vi "Poehali.vi"() -> (0 "?":string)   [LabVIEW 2016]
uses:
  Global 3.vi
panel:
  in  "Back":bool
  in  "?":bool
  out "2D Picture":picture
  # "Nice to meet you,  here,"
  # "You are at the Diversity orbital station. Here you can learn, create , grow and just \"dive into\" space exploration.\n        \n       Hope you will have fun !"
  # "ARE YOU READY ?"
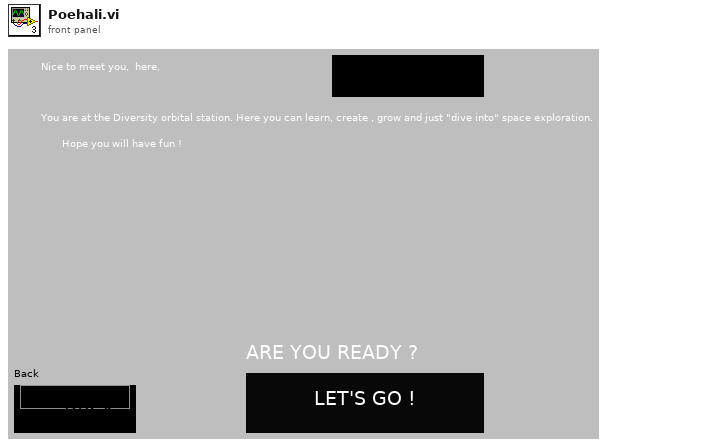
[diagram p1: front panel]
types:
  T1 = enum32{"Invalid", "Standard", "Closed", "Hidden", "Minimized", "Maximized"}
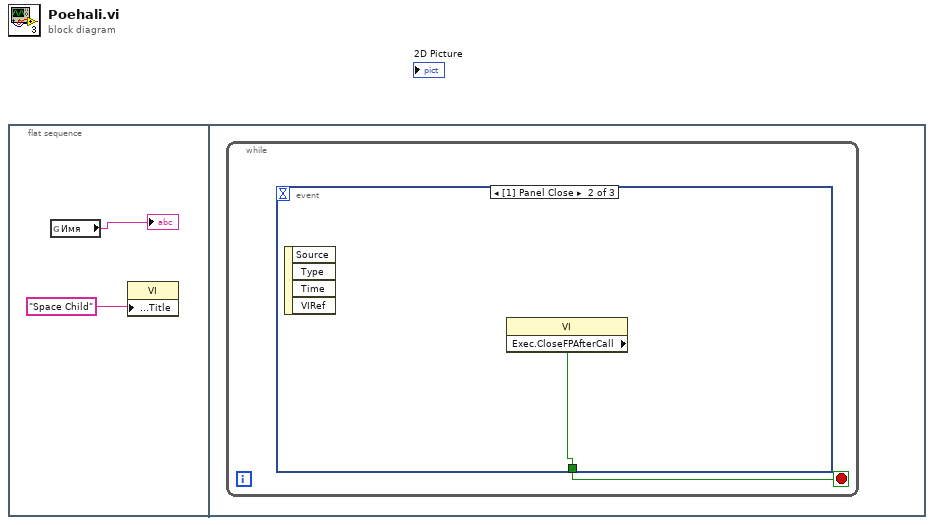
[diagram p0: block diagram]
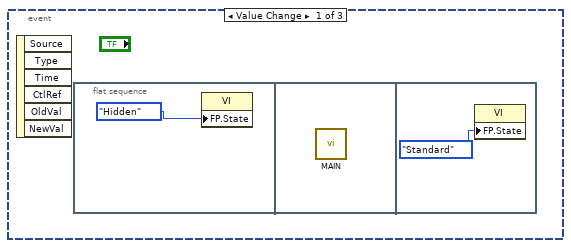
[diagram p2: hidden frame]
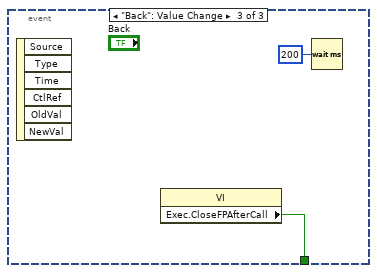
[diagram p3: hidden frame]
diagram:
  n1 = flat-sequence {
    frame #0 {
      n2 = global read "Global 3.vi" "Имя"() -> (→"?":string)
      n3 = property class="VI"("Front Panel.Title"="Space Child" ("Front Panel Window:Title")) -> ()  [unwired: 2 in, 2 out]
    }
    frame #1 {
      n4 = while {
        stop <- w3 stop-if-true
        n5 = event shown="[1] Panel Close" {
          selector: _ -> [_ _ _]
          dyn-events: _ -> [_ _ _]
          timeout: _ -> [_ _ _]
          tunnel: [_ w6 w8] -> w3
          event Value Change {
            n6 = event-data() -> ()  [unwired: 1 in, 6 out]
            n7 = flat-sequence {
              frame #0 {
                n8 = property class="VI"("FP.State"=T1."Hidden" ("Front Panel Window:State")) -> ()  [unwired: 2 in, 2 out]
              }
              frame #1 {
                n9 = call "MAIN.vi"() -> ()  [unwired: 2 in]
              }
              frame #2 {
                n10 = property class="VI"("FP.State"=T1."Standard" ("Front Panel Window:State")) -> ()  [unwired: 2 in, 2 out]
              }
            }
          }
          event Panel Close {
            n11 = event-data() -> ()  [unwired: 1 in, 4 out]
            n12 = property class="VI"() -> ("Exec.CloseFPAfterCall"=w6:bool)  [unwired: 2 in, 2 out]
          }
          event "Back": Value Change {
            n13 = event-data() -> ()  [unwired: 1 in, 6 out]
            n14 = property class="VI"() -> ("Exec.CloseFPAfterCall"=w8:bool)  [unwired: 2 in, 2 out]
            n15 = Wait (ms)(milliseconds to wait=u32 200) -> ()  [unwired: 1 out]
          }
        }
      }
    }
  }
